vi "FIR_2decimate_Filter0.vi"(8 "valid in":bool, 10 "Q in":fxp<+/-,16,14>, 11 "I in":fxp<+/-,16,14>) -> (0 "valid out":bool, 2 "Q out":fxp<+/-,16,14>, 3 "I out":fxp<+/-,16,14>)   [LabVIEW 2013]
uses:
  <vilib>/rvi/IPIntegrationNode/IPINode_Utilities/niFpgaIPINodeSimCore.vi
  <vilib>/rvi/XilinxIP/XIPIN_XNode/niFpgaXIPIN.xnode
  Filters/Polyphase filterbank decimate 2/Filter0/Decimate2Filter0_8B14D252B9D942A4BA762814218C3D7F.dll
  <vilib>/rvi/IPIntegrationNode/IPINode_Xnode/niFpgaIPINode.xnode
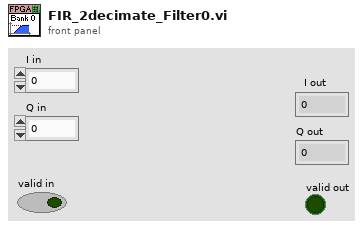
[diagram p1: front panel]
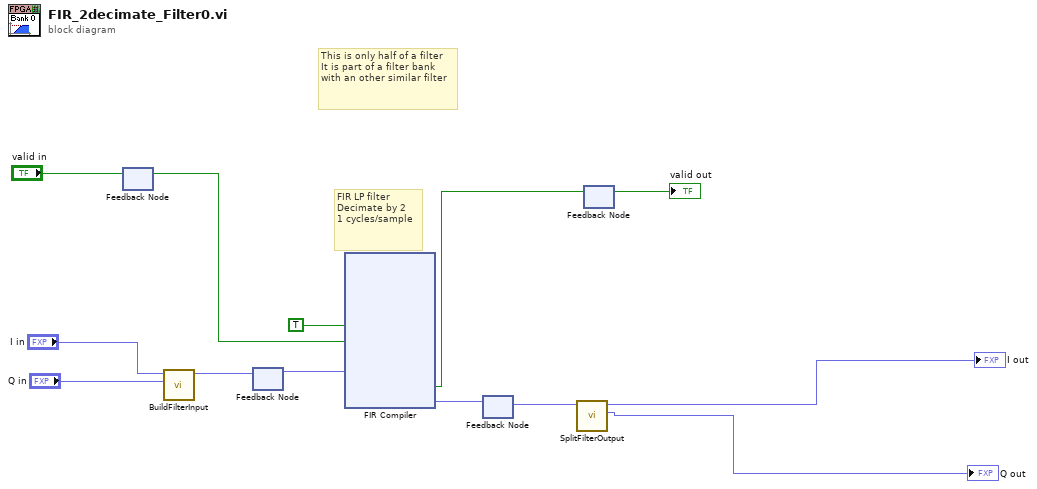
[diagram p0: block diagram]
diagram:
  # "This is only half of a filter\nIt is part of a filter bank\nwith an other similar filter"
  # "FIR LP filter\nDecimate by 2\n1 cycles/sample"
  n1 = feedback-in #1("valid in") -> ()
  n2 = feedback #1() -> (w7:bool)  [unwired: 1 in]
  n3 = call "BuildFilterInput.vi"("Q in"="Q in", "I in"="I in") -> ("Filter input"=w10:fxp<+,32,32>)  [unwired: 9 in]
  n4 = feedback-in #2(w10) -> ()
  n5 = feedback #2() -> (w6:fxp<+,32,32>)  [unwired: 1 in]
  n6 = xnode ("FIR Compiler")("aresetn"=TRUE, "s_axis_data_tvalid"=w7, "s_axis_data_tdata"=w6) -> ("m_axis_data_tvalid"=w5:bool, "m_axis_data_tdata"=w4:fxp<+,64,64>)  [unwired: 1 in, 1 out]
  n7 = feedback-in #3(w4) -> ()
  n8 = feedback #3() -> (w3:fxp<+,64,64>)  [unwired: 1 in]
  n9 = call "SplitFilterOutput.vi"("filter output"=w3) -> ("Q out"=→"Q out":fxp<+/-,16,14>, "I out"=→"I out":fxp<+/-,16,14>)  [unwired: 9 in]
  n10 = feedback-in #4(w5) -> ()
  n11 = feedback #4() -> (→"valid out":bool)  [unwired: 1 in]
